vi "Accelerometer.vi"() -> ()   [LabVIEW 2019]
uses:
  <vilib>/MakerHub/LINX/Public/Utilities/Open Serial.vi
  <vilib>/picture/3D Picture Control/Object/Create Object (drawable).vi
  <vilib>/picture/3D Picture Control/Object/Add Object (no reference).vi
  <vilib>/ErrorRing/Error Ring.xnode
  <vilib>/MakerHub/LINX/Public/Sensors/Accelerometer/ADXL345/ADXL345.lvlib
  <vilib>/MakerHub/LINX/LMH-LINX.lvlib
  <vilib>/picture/3D Picture Control/NI_3D Picture Control.lvlib
panel:
  in  "Ball":T1={"Red"=0.0, "Green"=0.0, "Blue"=1.0, "Alpha"=1.0}
  in  "Plate":T1={"Red"=1.0, "Green"=0.0, "Blue"=0.0, "Alpha"=1.0}
  in  "Angle":sgl=3.0
  out "3D Picture":refnum<vi>(3d-picture)
  out "Waveform Chart":T2(graph)
  in  "I2C Channel (0)":u8
  in  "Serial Port":refnum<visa-resource-name>="N/A"
  in  "stop":bool
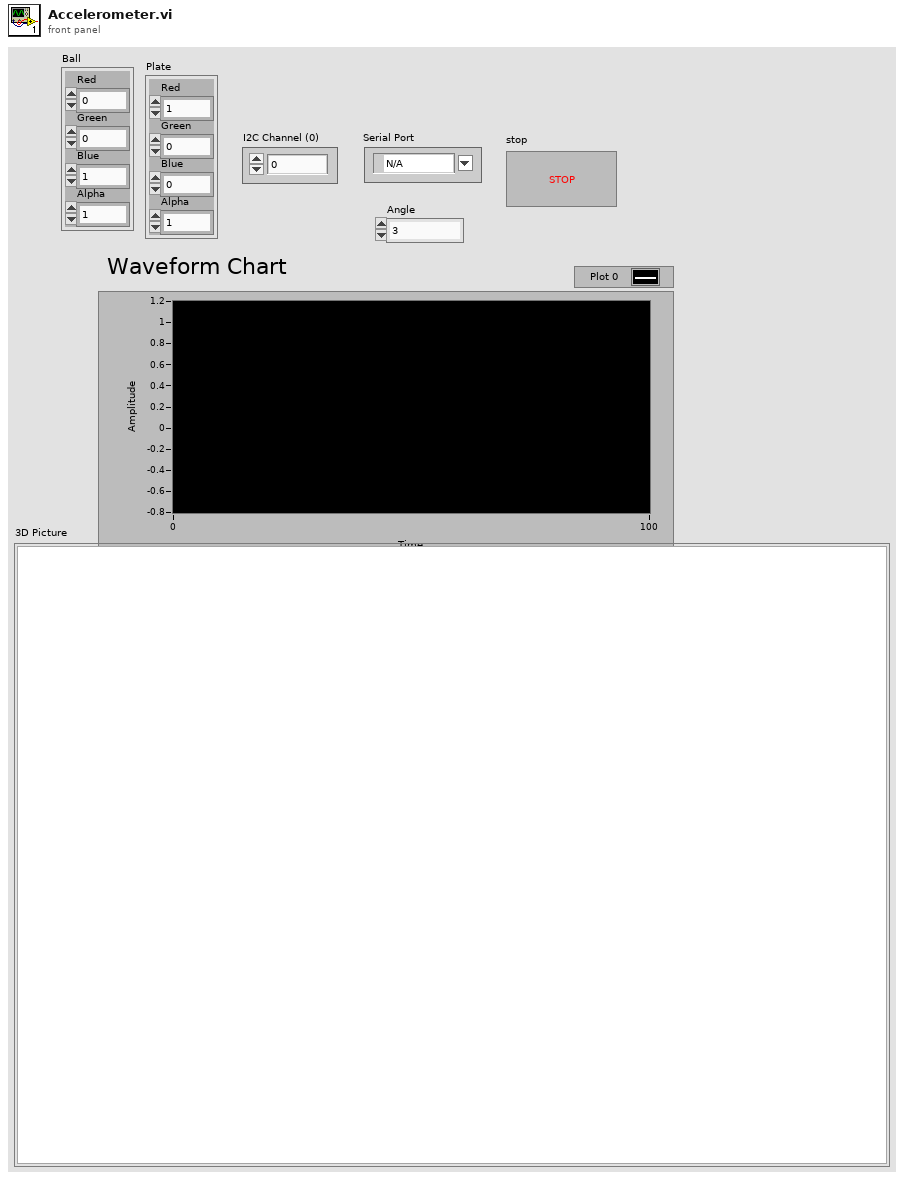
[diagram p1: front panel]
types:
  T1 = cluster{"Red":sgl, "Green":sgl, "Blue":sgl, "Alpha":sgl}
  T2 = cluster{"X Axis":dbl, "Y Axis":dbl, "Z Axis":dbl}
  T3 = typedef "LMH-LINX.lvlib/LINX Ref.ctl" = cluster{"IO":T4, "Interface":T5, "LINX Device Config":T6}
  T4 = typedef "LMH-LINX.lvlib/Platform.ctl" = enum16{"Remote", "Local"}
  T5 = typedef "LMH-LINX.lvlib/Interface.ctl" = enum16{"Serial", "TCP"}
  T6 = typedef "LMH-LINX.lvlib/Device.lvlib/LINX Device Config.ctl" = cluster{"Interface":T5, "COM Port":refnum<visa-resource-name>, "TCP Configuration":T7, "Device Family":u8, "Device ID":u8, "Device Name":string, "TCP Ref":refnum<k5>, "Channels":T8}
  T7 = typedef "LMH-LINX.lvlib/Device.lvlib/TCP Config.ctl" = cluster{"IP Address":string, "Port":u16}
  T8 = typedef "LMH-LINX.lvlib/Channels.ctl" = cluster{"DI":u8[], "DO":u8[], "AI":u8[], "AO":u8[], "PWM":u8[], "QE":u8[], "UART":u8[], "I2C 2":u8[], "SPI":u8[], "CAN":u8[], "Servo":u8[], "AI Ref (V)":dbl, "AI Resolution (Bits)":u8, "AO Ref (V)":dbl, "AO Resolution (Bits)":u8}
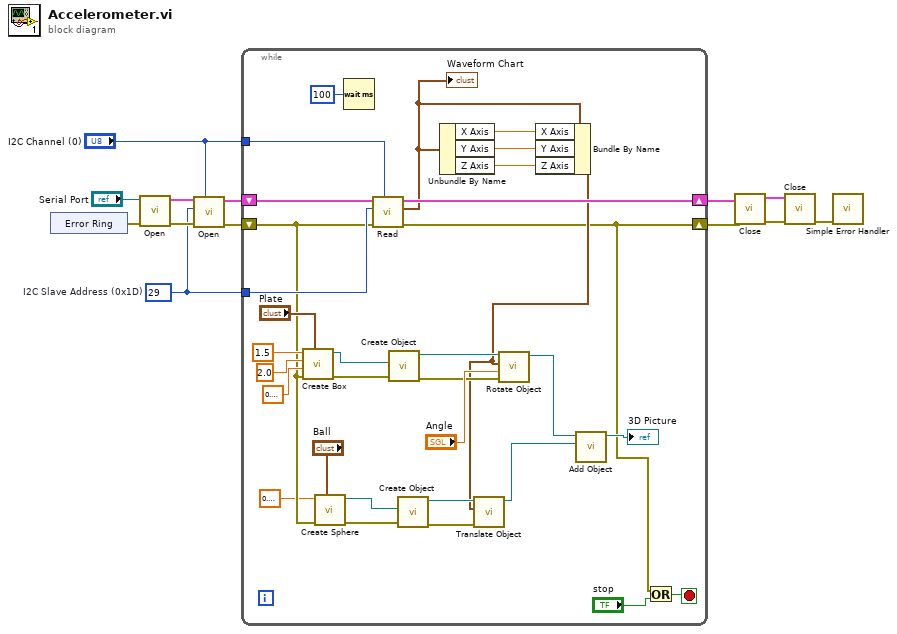
[diagram p0: block diagram]
diagram:
  w1 = u8 29  # I2C Slave Address (0x1D)
  n1 = xnode ("Error Ring")() -> ("error out"=w3:errorcluster)
  n2 = call-poly <vilib>:"Open.vi"("Error In"=w3, "Serial Port"="Serial Port") -> ("Error Out"=w7:errorcluster, "LINX Resource"=w10:T3)  [unwired: 7 in, 1 out]
  n3 = call <vilib>:"Open.vi"("I2C Channel (0)"="I2C Channel (0)", "Error In"=w7, "I2C Slave Address"=w1, "LINX Resource"=w10) -> ("Error Out"=w6:errorcluster, "LINX Resource"=w9:T3)  [unwired: 5 in, 1 out]
  n4 = while {
    tunnel: "I2C Channel (0)" -> [w41]
    tunnel: w1 -> [w40]
    shift-right: [w44] -> w8
    shift-left: w9 -> [w45]
    shift-right: [w14] -> w5
    shift-left: w6 -> [w25]
    stop <- w43 stop-if-true
    n5 = call <vilib>:"Create Box.vi"("Color"="Plate", "error in (no error)"=w25, "Length Z"=sgl 0.1, "Length Y"=sgl 2.0, "Length X"=sgl 1.5) -> ("error out"=w34:errorcluster, "New Box Refnum"=w35:refnum<vi>)  [unwired: 5 in]
    n6 = call <vilib>:"Create Sphere.vi"("Color"="Ball", "error in (no error)"=w25, "Radius"=sgl 0.2) -> ("error out"=w23:errorcluster, "New Sphere Refnum"=w24:refnum<vi>)  [unwired: 7 in]
    n7 = Wait (ms)(milliseconds to wait=u32 100) -> ()  [unwired: 1 out]
    n8 = call <vilib>:"Read.vi"("I2C Channel (0)"=w41, "Error In"=w25, "I2C Slave Address"=w40, "LINX Resource"=w45) -> ("Error Out"=w14:errorcluster, "Acceleration Data (g)"=w31:T2, "LINX Resource"=w44:T3)  [unwired: 5 in]
    "Waveform Chart" <- w31
    n9 = call-poly <vilib>:"Create Object.vi"("error in (no error)"=w34, "Geometry"=w35) -> ("error out"=w37:errorcluster, "Scene:New Object"=w36:refnum<vi>)  [unwired: 8 in]
    n10 = call-poly <vilib>:"Create Object.vi"("error in (no error)"=w23, "Geometry"=w24) -> ("error out"=w17:errorcluster, "Scene:New Object"=w18:refnum<vi>)  [unwired: 8 in]
    n11 = Unbundle By Name(w31) -> ("X Axis"=w30:dbl, "Y Axis"=w29:dbl, "Z Axis"=w32:dbl)
    n12 = Bundle By Name(cluster=w31, "X Axis"=w30, "Y Axis"=w29, "Z Axis"=w32) -> (w16:T2)
    n13 = call <vilib>:"Translate Object.vi"("error in (no error)"=w17, "Translation"=w16, "Scene.Object In"=w18) -> ("Scene.Object Out"=w15:refnum<vi>)  [unwired: 7 in, 1 out]
    n14 = call <vilib>:"Rotate Object.vi"("error in (no error)"=w37, "Angle"="Angle", "Axis"=w16, "Scene.Object In"=w36) -> ("Scene.Object Out"=w21:refnum<vi>)  [unwired: 6 in, 1 out]
    n15 = call-poly <vilib>:"Add Object.vi"("New Object In"=w15, "Scene Object In"=w21) -> ("Scene Object Out"=→"3D Picture":refnum<vi>)  [unwired: 8 in, 1 out]
    n16 = Or(x=w14, y="stop") -> (x .or. y?=w43:bool)
  }
  n17 = call <vilib>:"Close.vi"("Error In"=w5, "LINX Resource"=w8) -> ("Error Out"=w13:errorcluster, "LINX Resource"=w12:T3)  [unwired: 8 in]
  n18 = call <vilib>:"Close.vi"("Error In"=w13, "LINX Resource"=w12) -> ("Error Out"=w11:errorcluster)  [unwired: 9 in]
  n19 = call <vilib>:"Simple Error Handler.vi"("error in (no error)"=w11) -> ()  [unwired: 4 in, 5 out]
